vi "WebStartup.vi"(6 "LabVIEW Web Service":refnum<class "Web Service.lvclass">) -> ()   [LabVIEW 2015]
uses:
  <vilib>/wsapi/Web Service.lvclass
  TypeDef/RoomsActionEnum.ctl
panel:
  out "error out":errorcluster
  # "Use the web service input terminal to call the VIs on the Service subpalette of the Web Services palette. Do not remove it from the connector pane unless you don't need access to the palette."
  # "Any additional terminals added to the connector pane of a startup VI will be ignored."
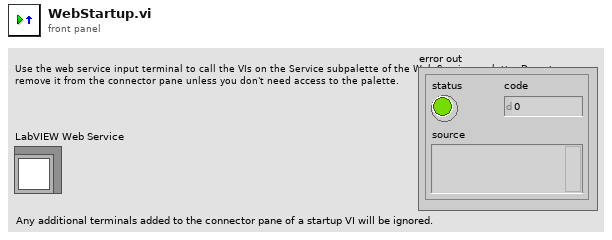
[diagram p1: front panel]
types:
  T1 = typedef "RoomsActionEnum.ctl" = enum16{"Init", "Add Room", "Remove Room", "Read Room", "Read Flag", "Read Flag State", "Write Flag State", "Read Flag Color", "Write Flag Color", "Read Bed Vacant", "Write Bed Vacant", "Read Personnel", "Add Personnel", "Remove Personnel", "Read Requests", "Add Request", "Remove Request", "Read Beacon ID", "Write Beacon ID", "Write Bed URL", "Read Bed URL", "Get Rooms Numbers"}
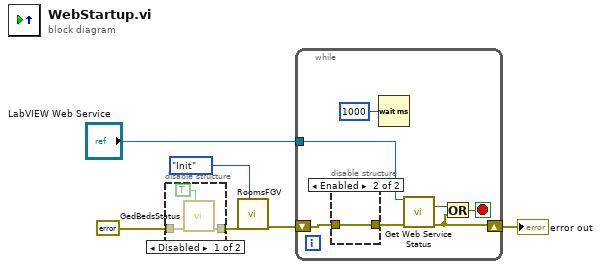
[diagram p0: block diagram]
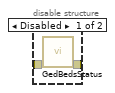
[diagram p3: hidden frame]
diagram:
  n1 = disable-structure shown="Disabled" {
    disable-tunnel: errorcluster {"status"=FALSE, "code"=0, "source"=""} ("error constant") -> [w9 w10]
    disable-tunnel: [w7 w10] -> w1
    frame Disabled {
      n2 = call "GedBedsStatus.vi"("Initialize"=TRUE, "error in (no error)"=w9) -> ("error out"=w7:errorcluster)  [unwired: 9 in]
    }
    frame Enabled {
    }
  }
  n3 = call "RoomsFGV.vi"("Actions"=RoomsActionEnum."Init", "error in (no error)"=w1) -> ("error out"=w4:errorcluster)  [unwired: 8 in, 1 out]
  n4 = while {
    tunnel: "LabVIEW Web Service" -> [w16]
    shift-right: [w14] -> w5
    shift-left: w4 -> [w12]
    stop <- w15 stop-if-true
    n5 = disable-structure shown="Enabled" {
      disable-tunnel: w12 -> [w19 w20]
      disable-tunnel: [w18 w20] -> w11
      frame Disabled {
        n6 = call "GedBedsStatus.vi"("error in (no error)"=w19) -> ("error out"=w18:errorcluster)  [unwired: 10 in]
      }
      frame Enabled {
      }
    }
    n7 = Wait (ms)(milliseconds to wait=u32 1000) -> ()  [unwired: 1 out]
    n8 = call <vilib>:"Get Web Service Status.vi"("LabVIEW Web Service"=w16, "error in (no error)"=w11) -> ("service stopping?"=w17:bool, "error out"=w14:errorcluster)  [unwired: 11 in, 1 out]
    n9 = Or(x=w17, y=w14) -> (x .or. y?=w15:bool)
  }
  "error out" <- w5
